vi "CtrlShutter_Init.vi"(8 "error in (no error)":errorcluster, 11 "VISA Refnum in":refnum<visa-resource-name>) -> (0 "error out":errorcluster, 2 "IDN":string, 3 "VISA Refnum out":refnum<visa-resource-name>)   [LabVIEW 2023]
uses:
  <vilib>/Instr/_visa.llb/VISA Configure Serial Port (Instr).vi
  <vilib>/Utility/error.llb/Error Cluster From Error Code.vi
  <vilib>/ErrorRing/Error Ring.xnode
panel:
  out "String":string
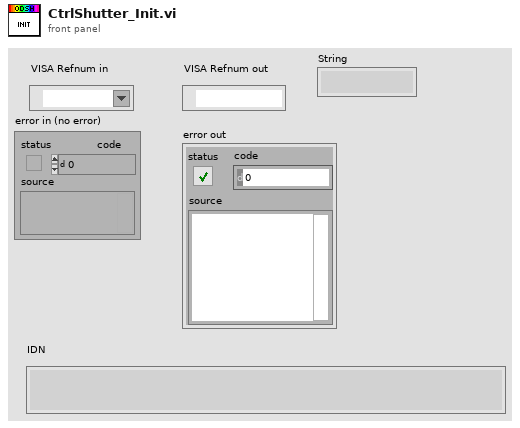
[diagram p1: front panel]
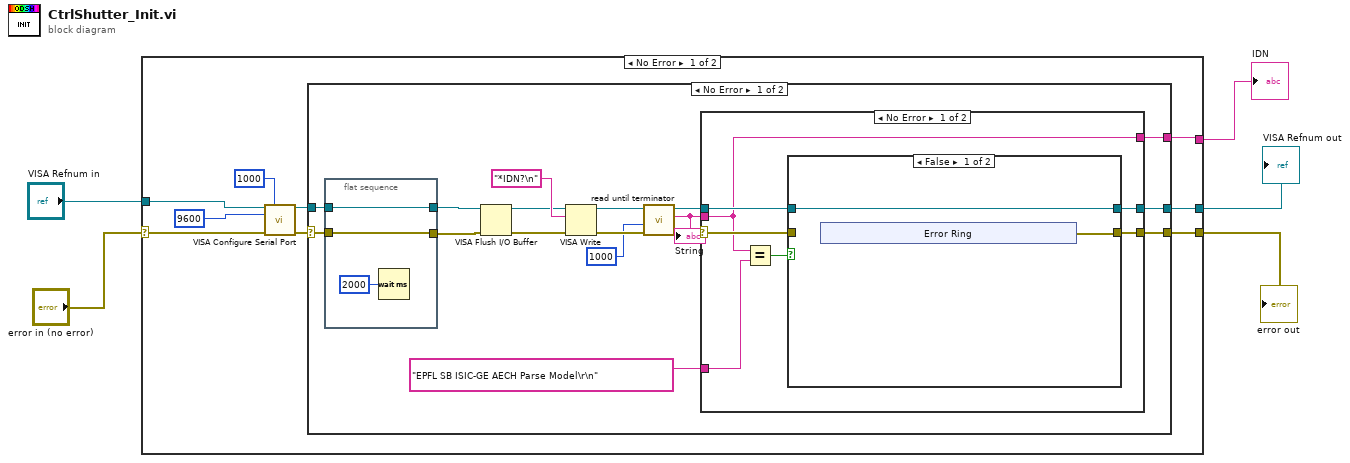
[diagram p0: block diagram]
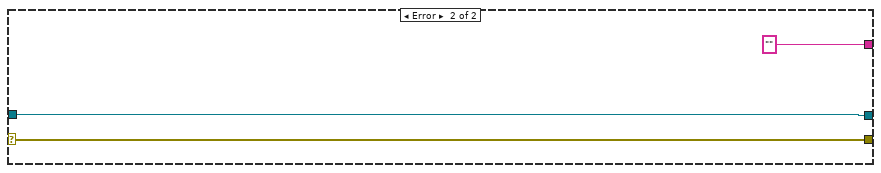
[diagram p4: hidden frame]
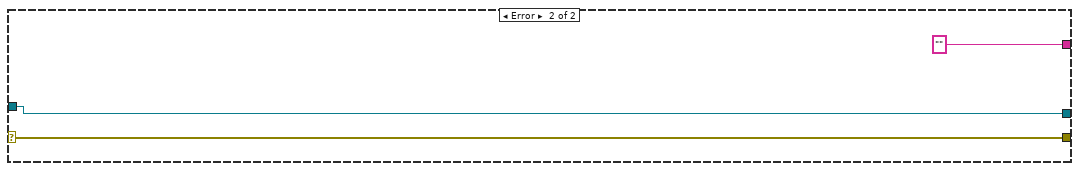
[diagram p5: hidden frame]
diagram:
  n1 = case shown="No Error" "error in (no error)" {
    selector: "error in (no error)" -> [w10 w59]
    tunnel: [w9 w58] -> w5
    tunnel: [w8 w59] -> w4
    tunnel: "VISA Refnum in" -> [w11 w58]
    tunnel: [w7 "" ("String")] -> w1
    frame No Error {
      n2 = call-poly "VISA Configure Serial Port"("VISA resource name"=w11, "timeout (10sec)"=u32 1000, "baud rate (9600)"=u32 9600, "error in (no error)"=w10) -> ("VISA resource name out"=w13:refnum<visa-resource-name>, "error out"=w6:errorcluster)  [unwired: 10 in]
      n3 = case shown="No Error" w6 {
        selector: w6 -> [w19 w56]
        tunnel: w13 -> [w24 w55]
        tunnel: [w22 w55] -> w9
        tunnel: [w21 w56] -> w8
        tunnel: [w17 "" ("String")] -> w7
        frame No Error {
          n4 = flat-sequence {
            tunnel: w24 -> [w51]
            tunnel: w19 -> [w52]
            tunnel: [w52] -> w26
            tunnel: [w51] -> w25
            frame #0 {
              n5 = Wait (ms)(milliseconds to wait=u32 2000) -> ()  [unwired: 1 out]
            }
          }
          n6 = VISA Flush I/O Buffer(VISA resource name=w25, error in (no error)=w26) -> (VISA resource name out=w27:refnum<visa-resource-name>, error out=w28:errorcluster)  [unwired: 1 in]
          n7 = VISA Write(VISA resource name=w27, write buffer="*IDN?\n", error in (no error)=w28) -> (VISA resource name out=w30:refnum<visa-resource-name>, error out=w16:errorcluster)  [unwired: 1 out]
          n8 = call "read until terminator.vi"("error in (no error)"=w16, "Timeout (ms)"=1000, "VISA Refnum in"=w30) -> ("error out"=w18:errorcluster, "String"=w20:string, "VISA Refnum out"=w23:refnum<visa-resource-name>)  [unwired: 6 in]
          "String" <- w20
          n9 = case shown="No Error" w18 {
            selector: w18 -> [w33 w50]
            tunnel: "EPFL SB ISIC-GE AECH Parse Model\r\n" ("y") -> [w38 _]
            tunnel: w23 -> [w37 w49]
            tunnel: [w36 w49] -> w22
            tunnel: [w35 w50] -> w21
            tunnel: w20 -> [w32 w48]
            tunnel: [w32 w48] -> w17
            frame No Error {
              n10 = Equal?(x=w32, y=w38) -> (x = y?=w34:bool)
              n11 = case shown="False" w34 {
                tunnel: w37 -> [w40 w47]
                tunnel: [w40 w47] -> w36
                tunnel: w33 -> [_ w46]
                tunnel: [w39 w46] -> w35
                frame False {
                  n12 = xnode "Error Ring"() -> ("error out"=w39:errorcluster)
                }
                frame True {
                }
              }
            }
            frame Error {
            }
          }
        }
        frame Error {
        }
      }
    }
    frame Error {
    }
  }
  "VISA Refnum out" <- w5
  "error out" <- w4
  "IDN" <- w1
